vi "Get 1D Array Double Complex.vi"(5 "use temporary file? (F)":bool, 7 "data type of variable":cdb[](array[numeric]), 8 "error in":errorcluster, 10 "variable name":string, 11 "GOLPI ref. in":T1={"pipe handle"={"lv_proc.dll file path"=path "", "process instance handle"=[]}, "fast read timeout [ms]"=500, "fast read settle time [ms]"=10, "fast read to multiple [ms]"=1, "max elements per input line"=100, "slow read timeout [ms]"=5000, "stdin double format specifier"="%_16e", "max elements per stdout output column"=100}) -> (0 "error out":errorcluster, 2 "value":cdb[](array[numeric]) format="%.2f", 3 "GOLPI ref. out":T1={"pipe handle"={"lv_proc.dll file path"=path "", "process instance handle"=[]}, "fast read timeout [ms]"=500, "fast read settle time [ms]"=10, "fast read to multiple [ms]"=1, "max elements per input line"=100, "slow read timeout [ms]"=5000, "stdin double format specifier"="%_16e", "max elements per stdout output column"=100})   [LabVIEW 2013, in "GOLPI library.lvlib"]
doc: "Part of polymorph Get Variable.vi"
uses:
  GOLPI library.lvlib
  Type Definitions/Custom Error Codes Enum Type Def.vi
  LV Process.lvlibp/Pipe Handle.ctl
  LV Process.lvlibp
  Type Definitions/GOLPI reference Type Def.ctl
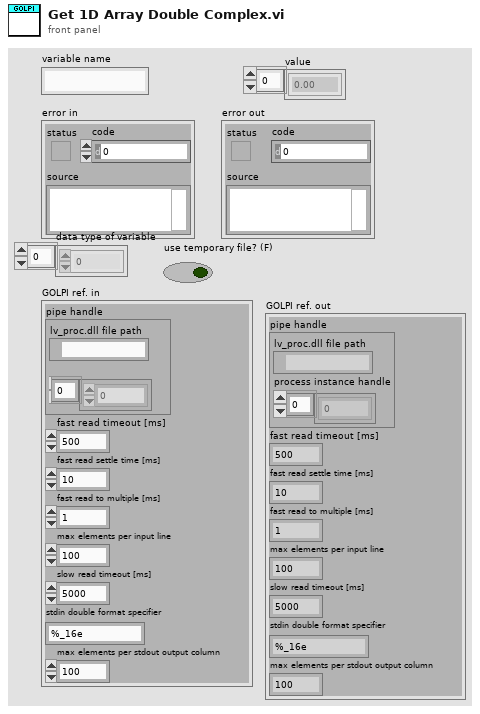
[diagram p1: front panel]
types:
  T1 = typedef "GOLPI library.lvlib/GOLPI reference Type Def.ctl" = cluster{"pipe handle":T2, "fast read timeout [ms]":u32, "fast read settle time [ms]":u32, "fast read to multiple [ms]":u32, "max elements per input line":u32, "slow read timeout [ms]":u32, "stdin double format specifier":string, "max elements per stdout output column":u32}
  T2 = typedef "LV Process.lvlibp/Pipe Handle.ctl" = cluster{"lv_proc.dll file path":path, "process instance handle":u32[]}
  T3 = typedef "GOLPI library.lvlib/Custom Error Codes Enum Type Def.vi" = enum16{"no error", "00 working directory PAR1 missing", "01 octave binary PAR1 missing", "02 octave report error PAR1", "03 empty output last cmd PAR1", "04 missing temporary file PAR1", "05 pwd PAR 1 not exist", "10 var PAR1 not string, vect", "11 var PAR1 not num, scal, ~compl", "12 var PAR1 not num, scal, compl", "13 var PAR1 not num, vect, ~compl", "14 var PAR1 not num, vect, compl", "15 var PAR1 not num, mat, ~compl", "16 var PAR1 not num, mat, ~compl", "30 WARNING read timeout", "99 not finished"}
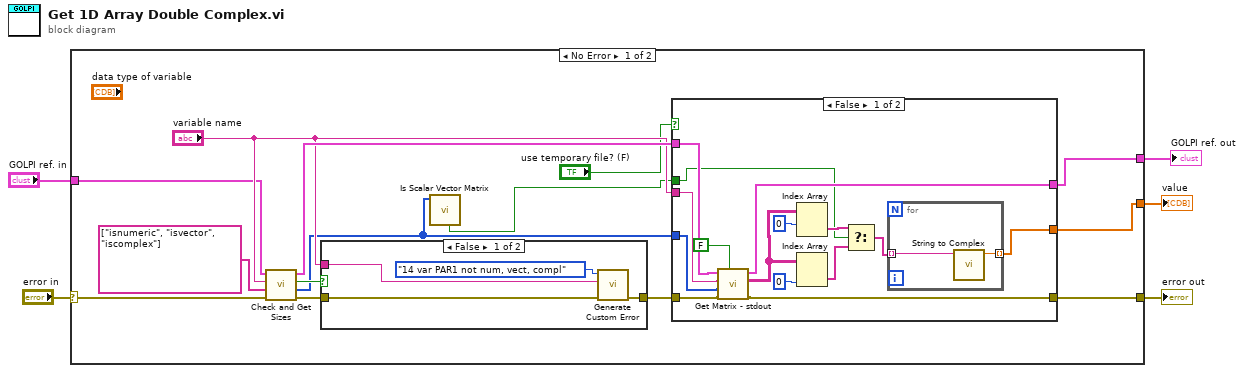
[diagram p0: block diagram]
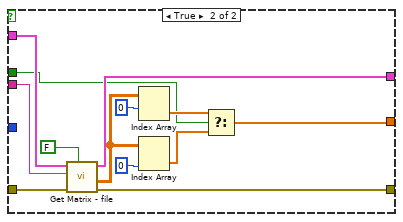
[diagram p2: hidden frame]
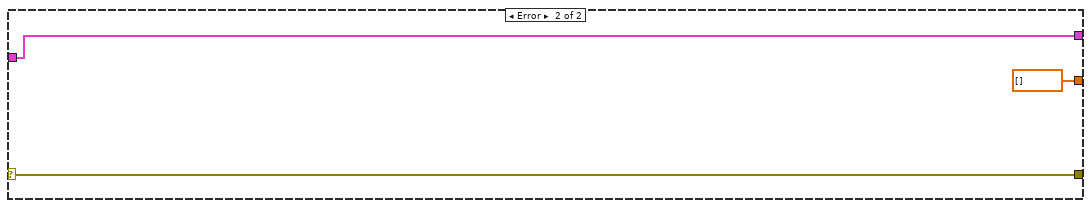
[diagram p4: hidden frame]
diagram:
  n1 = case shown="No Error" "error in" {
    selector: "error in" -> [w18 w57]
    tunnel: [w13 w57] -> w5
    tunnel: [w11 cdb[] [] ("value")] -> w3
    tunnel: "GOLPI ref. in" -> [w7 w55]
    tunnel: [w6 w55] -> w1
    frame No Error {
      n2 = call "Check and Get Sizes.vi"("error in (no error)"=w18, "test commands"=string[] ["isnumeric", "isvector", "iscomplex"], "variable name"="variable name", "GOLPI ref. in"=w7) -> ("error out"=w17:errorcluster, "octave sizes"=w9:i32[], "all tests OK?"=w19:bool, "GOLPI ref. out"=w15:T1)  [unwired: 4 in]
      n3 = case shown="False" w19 {
        tunnel: w17 -> [w52 w54]
        tunnel: [w51 w54] -> w14
        tunnel: "variable name" -> [w50 _]
        frame False {
          n4 = call "Generate Custom Error.vi"("error in"=w52, "PAR1"=w50, "GOLPI error"=Custom_Error_Codes_Enum_Type_Def.vi."14 var PAR1 not num, vect, compl" ("Enum")) -> ("error out"=w51:errorcluster)  [unwired: 8 in]
        }
        frame True {
        }
      }
      n5 = call "Is Scalar Vector Matrix.vi"("octave sizes"=w9) -> ("row vector?"=w8:bool)  [unwired: 5 in, 5 out]
      n6 = case shown="False" "use temporary file? (F)" {
        tunnel: w15 -> [w34 w41]
        tunnel: [w33 w42] -> w6
        tunnel: w14 -> [w31 w44]
        tunnel: [w32 w43] -> w13
        tunnel: w9 -> [w30 _]
        tunnel: w8 -> [w20 w37]
        tunnel: "variable name" -> [w29 w38]
        tunnel: [w27 w39] -> w11
        frame False {
          n7 = call "Get Matrix - stdout.vi"("is string"=FALSE, "error in (no error)"=w31, "octave sizes"=w30, "variable name"=w29, "GOLPI ref. in"=w34) -> ("error out"=w32:errorcluster, "array"=w21:string[][], "GOLPI ref. out"=w33:T1)  [unwired: 4 in]
          n8 = Index Array(array=w21, index (row)=0) -> (element=w24:string[])  [unwired: 1 in]
          n9 = Index Array(array=w21, index (col)=0 ("disabled index (col)")) -> (element=w23:string[])  [unwired: 1 in]
          n10 = Select(t=w24, s=w20, f=w23) -> (s? t:f=w22:string[])
          n11 = for {
            tunnel: w22 -> [w36] mode=indexing
            tunnel: [w35] -> w27 mode=indexing
            n12 = call "String to Complex.vi"("string"=w36) -> ("complex number"=w35:cdb)  [unwired: 10 in]
          }
        }
        frame True {
          n13 = call "Get Matrix - file.vi"("is string"=FALSE, "error in (no error)"=w44, "variable name"=w38, "GOLPI ref. in"=w41) -> ("error out"=w43:errorcluster, "cmplx double array"=w40:cdb[][], "GOLPI ref. out"=w42:T1)  [unwired: 3 in, 2 out]
          n14 = Index Array(array=w40, index (row)=0) -> (element=w47:cdb[])  [unwired: 1 in]
          n15 = Index Array(array=w40, index (col)=0 ("disabled index (col)")) -> (element=w46:cdb[])  [unwired: 1 in]
          n16 = Select(t=w47, s=w37, f=w46) -> (s? t:f=w39:cdb[])
        }
      }
    }
    frame Error {
    }
  }
  "value" <- w3
  "error out" <- w5
  "GOLPI ref. out" <- w1
